vi "Write Data.vi"(8 "error in (no error)":errorcluster, 10 "Data":T1[](array[typedef]), 11 "Log Message in":refnum<class "Log Message.lvclass">) -> (0 "error out":errorcluster, 3 "Log Message out":refnum<class "Log Message.lvclass">)   [LabVIEW 2024, in "AIM ARINC 429 Engine.lvlib" / "Implementation.lvlib" / "Word Logging.lvlib" / "Log Message.lvclass"]
uses:
  Log Message.lvclass
  Word.ctl
  Log Message.lvclass/Log Message.ctl
  Implementation.lvlib
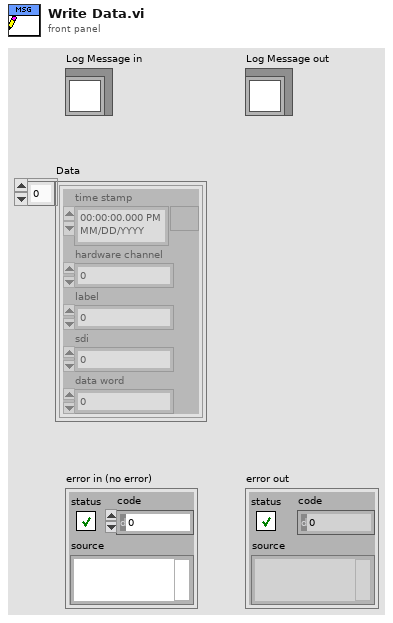
[diagram p1: front panel]
types:
  T1 = typedef "AIM ARINC 429 Engine.lvlib/Implementation.lvlib/Word.ctl" = cluster{"time stamp":timestamp, "hardware channel":u8, "label":u8, "sdi":u8, "data word":u32}
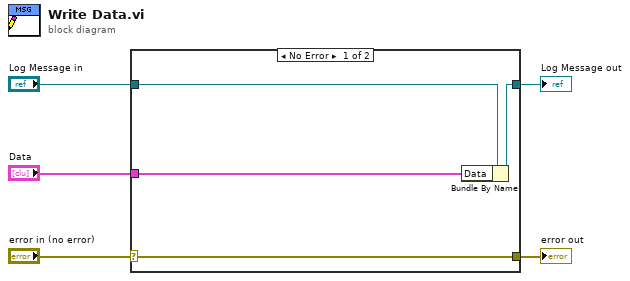
[diagram p0: block diagram]
diagram:
  n1 = case shown="No Error" "error in (no error)" {
    selector: "error in (no error)" -> [w9 w10]
    tunnel: [w9 w10] -> w4
    tunnel: [w7 w11] -> w2
    tunnel: "Log Message in" -> [w8 w11]
    tunnel: "Data" -> [w6 _]
    frame No Error {
      n2 = Bundle By Name(cluster=w8, "Data"=w6) -> (w7:refnum<class "Log Message.lvclass">)
    }
    frame Error {
    }
  }
  "error out" <- w4
  "Log Message out" <- w2
